vi "Create Stem.vi"(6 "Draw Mode":T9(ring)=enum."Triangles", 7 "3D Stem Property":T4={"General Property"={"Plot Name"="", "Coordinate System"=enum."Cartesian", "Opacity"=0.0}, "Projection Property"={"Draw XY"=FALSE, "Draw YZ"=FALSE, "Draw XZ"=FALSE}, "Plot Property"={"Sprite Type"=enum."Empty Square", "Point Size"=0.0, "Color Ramp Cluster"={"Color Ramp Style"=enum."None", "Color Ramp Array"=[16711934, 393471, 57855, 4390754, 16449346, 16744722, 16711680], "Color Ramp Index"=[45, 91, 133, 175, 219, 255], "Interpolate?"=FALSE, "Logarithm?"=FALSE}, "Line Style"=enum."None", "Line Width"=0.0, "Line Color"=0, "Antialiasing"=FALSE}}, 8 "error in (no error)":errorcluster, 9 "Actual Transform In":T8, 10 "Plot Representation In":T1, 11 "Plot Object In":refnum<vi>) -> (0 "error out":errorcluster, 1 "Actual Transform Out":T8, 2 "Plot Representation Out":T1, 3 "Plot Object Out":refnum<vi>, 4 "Stem Object Out":refnum<vi>)   [LabVIEW 2020, in "3D Stem.lvclass"]
uses:
  <vilib>/Math Plots/3D Math Plots/3D Stem/3D Stem/3D Stem.lvclass
  <vilib>/Math Plots/3D Math Plots/3D Plot/3D Plot/Typedef/Actual Transform.ctl
  <vilib>/Math Plots/3D Math Plots/3D Plot/3D Plot/Typedef/Range Clusters.ctl
  <vilib>/Math Plots/3D Math Plots/3D Plot/3D Plot/Typedef/Plot Representation.ctl
  <vilib>/Math Plots/3D Math Plots/3D Plot/3D Plot/Typedef/Mesh Data.ctl
  <vilib>/Math Plots/3D Math Plots/3D Stem/3D Stem/Typedef/3D Stem Property.ctl
  <vilib>/Math Plots/3D Math Plots/3D Plot/3D Plot/Typedef/Sprite Type.ctl
  <vilib>/Math Plots/3D Math Plots/3D Plot/3D Plot/Typedef/Color Ramp Cluster.ctl
  <vilib>/Math Plots/3D Math Plots/3D Plot/3D Plot/Typedef/Line Type.ctl
  <vilib>/Utility/miscctls.llb/LV3DPointTypeDef.ctl
  <vilib>/picture/3D Picture Control/NI_3D Picture Control.lvlib
  <vilib>/Math Plots/3D Math Plots/3D Plot/3D Plot/3D Plot.lvclass
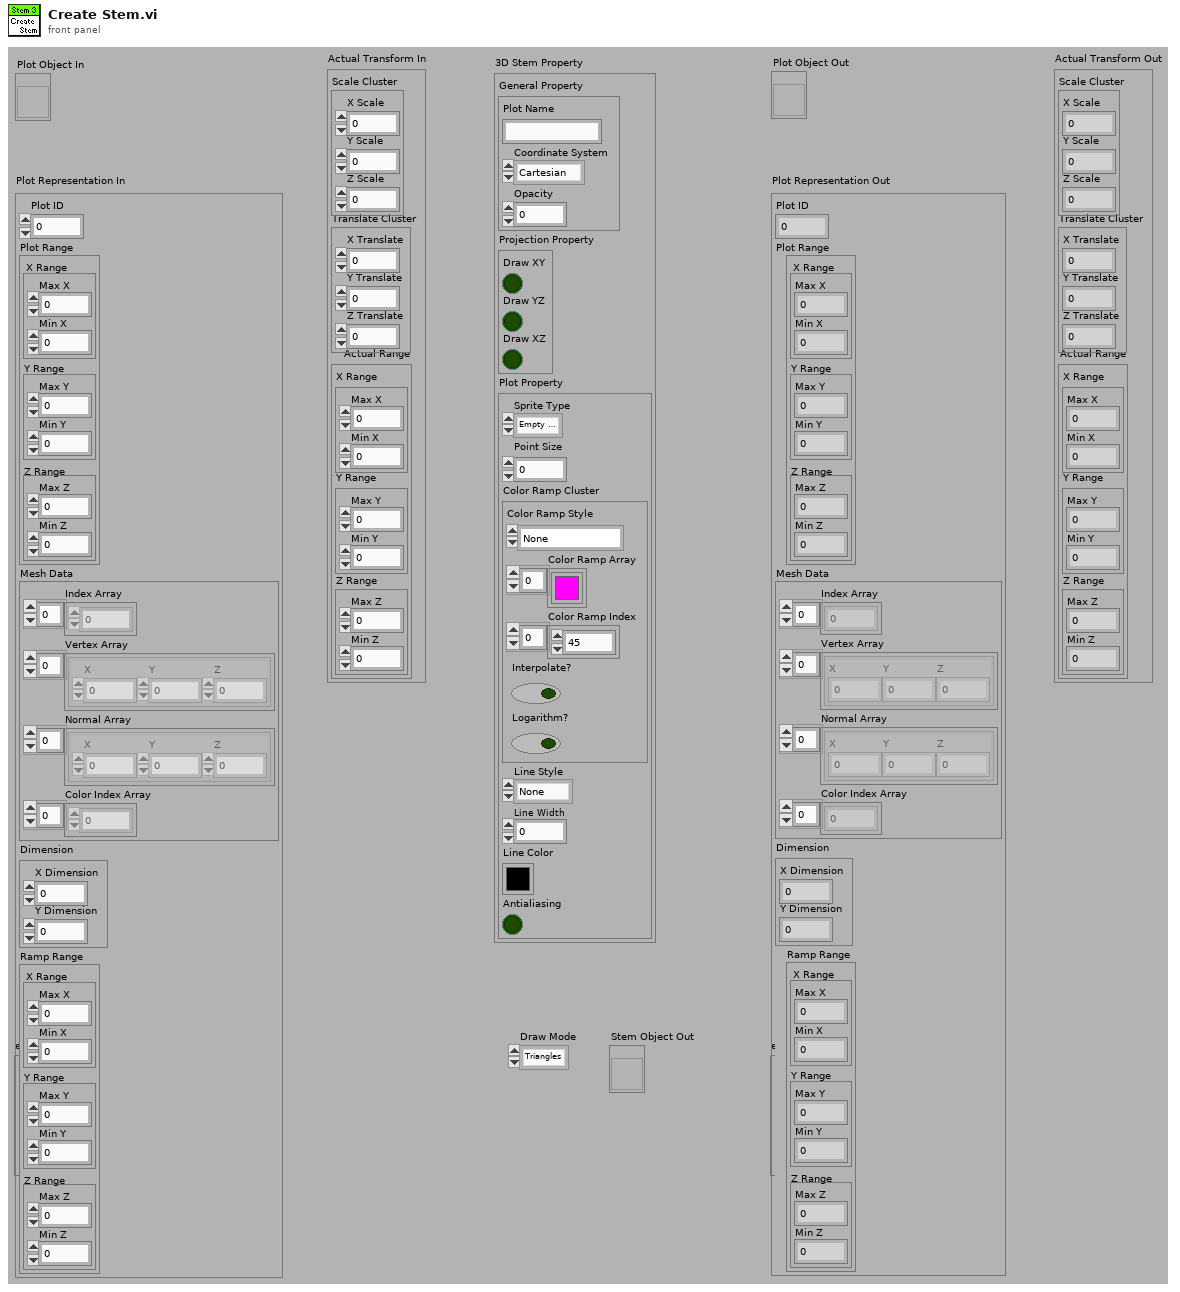
[diagram p1: front panel]
types:
  T1 = typedef "3D Plot.lvclass/Plot Representation.ctl" = cluster{"Plot ID":i32, "Plot Range":T2, "Mesh Data":T3, "Dimension":cluster{"X Dimension":i32, "Y Dimension":i32}, "Ramp Range":T2}
  T2 = typedef "3D Plot.lvclass/Range Clusters.ctl" = cluster{"X Range":cluster{"Max X":sgl, "Min X":sgl}, "Y Range":cluster{"Max Y":sgl, "Min Y":sgl}, "Z Range":cluster{"Max Z":sgl, "Min Z":sgl}}
  T3 = typedef "3D Plot.lvclass/Mesh Data.ctl" = cluster{"Index Array":u32[], "Vertex Array":cluster{"X":sgl, "Y":sgl, "Z":sgl}[], "Normal Array":cluster{"X":sgl, "Y":sgl, "Z":sgl}[], "Color Index Array":i32[]}
  T4 = typedef "3D Stem.lvclass/3D Stem Property.ctl" = cluster{"General Property":cluster{"Plot Name":string, "Coordinate System":enum16{"Cartesian", "Cylindrical", "Spherical"}, "Opacity":sgl}, "Projection Property":cluster{"Draw XY":bool, "Draw YZ":bool, "Draw XZ":bool}, "Plot Property":cluster{"Sprite Type":T5, "Point Size":sgl, "Color Ramp Cluster":T6, "Line Style":T7, "Line Width":sgl, "Line Color":u32, "Antialiasing":bool}}
  T5 = typedef "3D Plot.lvclass/Sprite Type.ctl" = enum16{"None", "Empty Square", "Solid Square", "Empty Diamond", "Solid Diamond", "Empty Circle", "Solid Circle", "Asterisk", "Bold X", "Wireframe Sphere", "Solid Sphere", "Wireframe Cube", "Solid Cube"}
  T6 = typedef "3D Plot.lvclass/Color Ramp Cluster.ctl" = cluster{"Color Ramp Style":enum16{"None", "Shaded", "Color spectrum", "Grey scale", "Custom"}, "Color Ramp Array":u32[], "Color Ramp Index":i32[], "Interpolate?":bool, "Logarithm?":bool}
  T7 = typedef "3D Plot.lvclass/Line Type.ctl" = enum16{"None", "Solid", "Dash", "Dot", "Dash Dot"}
  T8 = typedef "3D Plot.lvclass/Actual Transform.ctl" = cluster{"Scale Cluster":cluster{"X Scale":sgl, "Y Scale":sgl, "Z Scale":sgl}, "Translate Cluster":cluster{"X Translate":sgl, "Y Translate":sgl, "Z Translate":sgl}, "Actual Range":T2}
  T9 = enum16{"Points", "Lines", "Line Strip", "Line Loop", "Triangles", "Triangle Strip", "Triangle Fan", "Quads", "Quad Strip", "Polygon"}
  T10 = typedef "LV3DPointTypeDef.ctl" = cluster{"X":sgl, "Y":sgl, "Z":sgl}
  T11 = enum16{"Overall", "Per Primitive", "Per Vertex", "Binding Off"}
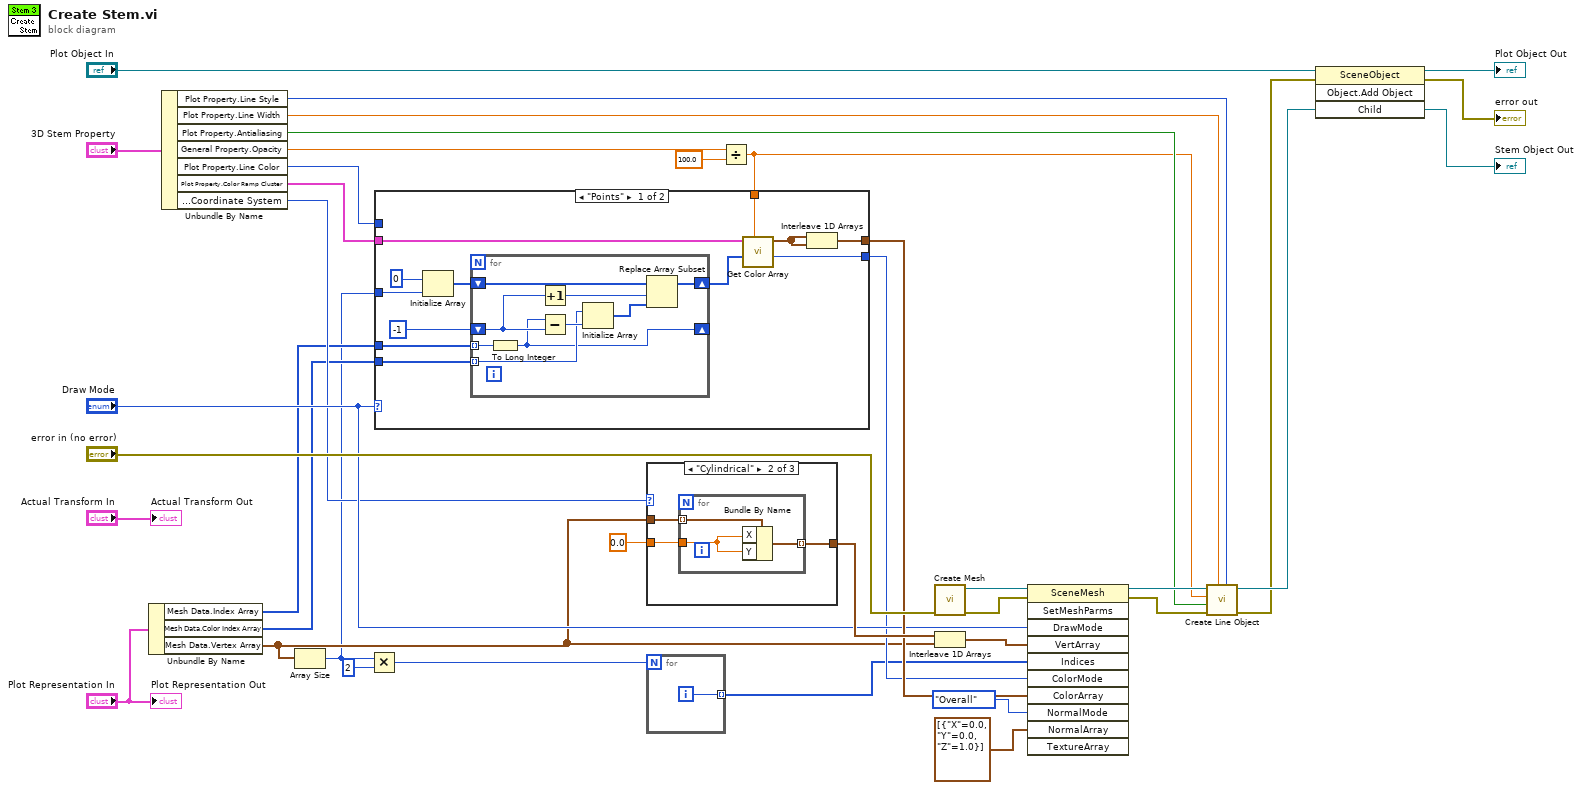
[diagram p0: block diagram]
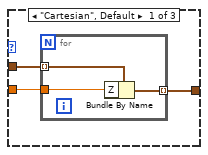
[diagram p2: hidden frame]
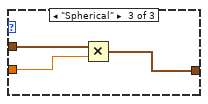
[diagram p3: hidden frame]
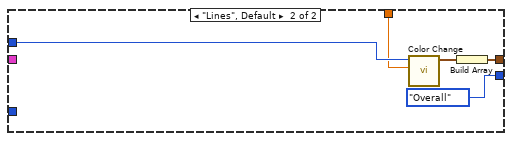
[diagram p4: hidden frame]
diagram:
  n1 = Unbundle By Name("Plot Representation In") -> ("Mesh Data.Index Array"=w3:u32[], "Mesh Data.Color Index Array"=w2:i32[], "Mesh Data.Vertex Array"=w7:cluster{"X":sgl, "Y":sgl, "Z":sgl}[])
  n2 = Unbundle By Name("3D Stem Property") -> ("Plot Property.Line Style"=w13:T7, "Plot Property.Line Width"=w14:sgl, "Plot Property.Antialiasing"=w11:bool, "General Property.Opacity"=w12:sgl, "Plot Property.Line Color"=w26:u32, "Plot Property.Color Ramp Cluster"=w22:T6, "General Property.Coordinate System"=w15:enum16{"Cartesian", "Cylindrical", "Spherical"})
  n3 = Array Size(array=w7) -> (size(s)=w1:i32)
  n4 = Multiply(x=w1, y=2) -> (x*y=w5:i32)
  n5 = case shown="\"Cylindrical\"" w15 {
    tunnel: [w41 w46 w52] -> w28
    tunnel: w7 -> [w40 w47 w53]
    tunnel: sgl 0.0 ("X") -> [w39 w45 w51]
    frame "Cartesian", Default {
      n6 = for {
        tunnel: w40 -> [w44] mode=indexing
        tunnel: [w43] -> w41 mode=indexing
        tunnel: w39 -> [w42]
        n7 = Bundle By Name(cluster=w44, "Z"=w42) -> (w43:cluster{"X":sgl, "Y":sgl, "Z":sgl})
      }
    }
    frame "Cylindrical" {
      n8 = for {
        tunnel: w47 -> [w50] mode=indexing
        tunnel: [w49] -> w46 mode=indexing
        tunnel: w45 -> [w48]
        n9 = Bundle By Name(cluster=w50, "X"=w48, "Y"=w48) -> (w49:cluster{"X":sgl, "Y":sgl, "Z":sgl})
      }
    }
    frame "Spherical" {
      n10 = Multiply(x=w53, y=w51) -> (x*y=w52:cluster{"X":sgl, "Y":sgl, "Z":sgl}[])
    }
  }
  n11 = for {
    N: w5 -> [_]
    tunnel: [w54] -> w4 mode=indexing
    i -> [w54]
  }
  n12 = Divide(x=w12, y=sgl 100.0) -> (x/y=w10:sgl)
  n13 = case shown="\"Points\"" "Draw Mode" {
    tunnel: w26 -> [_ w80]
    tunnel: [w64 w78] -> w25
    tunnel: w10 -> [w63 w77]
    tunnel: [w66 T11."Overall" ("Color Binding Mode")] -> w23
    tunnel: w22 -> [w62 _]
    tunnel: w3 -> [w58 _]
    tunnel: w2 -> [w57 _]
    tunnel: w1 -> [w56 _]
    frame "Points" {
      n14 = Initialize Array(0, w56) -> (w60:i32[])
      n15 = for {
        tunnel: w58 -> [w69] mode=indexing
        tunnel: w57 -> [w74] mode=indexing
        shift-right: [w72] -> w59
        shift-left: w60 -> [w73]
        shift-right: [w68] -> _
        shift-left: -1 -> [w70]
        n16 = To Long Integer(number=w69) -> (32bit integer=w68:i32)
        n17 = Increment(x=w70) -> (x+1=w67:i32)
        n18 = Subtract(x=w68, y=w70) -> (x-y=w75:i32)
        n19 = Initialize Array(w74, w75) -> (w71:i32[])
        n20 = Replace Array Subset(array=w73, new element=w71, index=w67) -> (w72:i32[])
      }
      n21 = call <vilib>:"Get Color Array.vi"("Alpha"=w63, "Color Index Array"=w59, "Color Ramp Cluster"=w62) -> ("Color Binding Mode"=w66:T11, "Color Array"=w65:cluster{"R":sgl, "G":sgl, "B":sgl, "A":sgl}[])  [unwired: 3 in, 4 out]
      n22 = Interleave 1D Arrays(w65, w65) -> (w64:cluster{"R":sgl, "G":sgl, "B":sgl, "A":sgl}[])
    }
    frame "Lines", Default {
      n23 = call <vilib>:"Color Change.vi"("Alpha"=w77, "Color"=w80) -> ("RGBA"=w79:cluster{"R":sgl, "G":sgl, "B":sgl, "A":sgl})  [unwired: 9 out]
      n24 = Build Array(w79) -> (w78:cluster{"R":sgl, "G":sgl, "B":sgl, "A":sgl}[])
    }
  }
  n25 = call <vilib>:"Create Mesh.vi"("error in (no error)"="error in (no error)") -> ("error out"=w30:errorcluster, "New Mesh Refnum"=w32:refnum<vi>)  [unwired: 9 out]
  n26 = Interleave 1D Arrays(w28, w7) -> (w27:cluster{"X":sgl, "Y":sgl, "Z":sgl}[])
  n27 = invoke class="SceneMesh" method="SetMeshParms"(reference=w32, error in=w30, "DrawMode"="Draw Mode", "VertArray"=w27, "Indices"=w4, "ColorMode"=w23, "ColorArray"=w25, "NormalMode"=T11."Overall" ("Normal Binding Mode"), "NormalArray"=T10[] [{"X"=0.0, "Y"=0.0, "Z"=1.0}] ("Normal Array")) -> (reference out=w20:refnum<vi>, error out=w19:errorcluster)  [unwired: 2 in, 9 out]
  n28 = call <vilib>:"Create Line Object.vi"("Line Style"=w13, "Line Width"=w14, "error in (no error)"=w19, "Antialiasing"=w11, "Alpha"=w10, "Mesh Ref In"=w20) -> ("error out"=w16:errorcluster, "Object Ref Out"=w18:refnum<vi>)  [unwired: 4 out]
  n29 = invoke class="SceneObject" method="Object.Add Object"(reference="Plot Object In", error in=w16, "Child"=w18) -> (reference out=→"Plot Object Out":refnum<vi>, error out=→"error out":errorcluster, "Child"=→"Stem Object Out":refnum<vi>)  [unwired: 1 in, 1 out]
  "Actual Transform Out" <- "Actual Transform In"
  "Plot Representation Out" <- "Plot Representation In"
